vi "IMU AHRS Demo.vi"() -> ()   [LabVIEW 2014]
doc: "This example shows how to move a motor connected to an encoder and a wheel, and then read information about the system from an encoder.\n\nThis is an example of how to use feedback (from the encoder) to create an open loop system. If some control method was used, for example using PID, a closed loop system could be created."
uses:
  <vilib>/Rock Robotics/SystemInterfaces/i2clib/i2c_bus.ctl
  <vilib>/Platform/TimedLoop/XDataNode/timing_clust.ctl
  <vilib>/Platform/TimedLoop/XDataNode/nitl_modes.ctl
  <vilib>/Platform/TimedLoop/XDataNode/wakeup.ctl
  <vilib>/platform/TimedLoop/XDataNode/XDataNode.xnode
  <vilib>/Platform/TimedLoop/XDataNode/XDNodeRunTimeDep.lvlib
panel:
  out "R/P Alpha":dbl
  out "Yaw Alpha":dbl
  out "BadCal Mag":bool
  in  "I2C Bus":T1
  out "Anomaly":bool
  in  "Mag Set":T2={"Data Rate"=enum."220 Hz", "Range"=1, "Sense Enable"=TRUE, "Mag Scale"={"Xscale"=1.0, "Yscale"=1.0, "Zscale"=1.0}, "Mag Offset"={"Xzero"=0.0, "Yzero"=0.0, "Zzero"=0.0}, "Anomaly Thresh"=2.4, "Local Mag"=48.0} {"Range" items=["+/- 130 uT"=1, "+/- 190 uT"=2, "+/- 250 uT"=3, "+/- 400 uT"=4, "+/- 470 uT"=5, "+/- 560 uT"=6, "+/- 810 uT"=7]}
  out "Roll":cluster{dbl, dbl}(knob)={0.0, 152.0639793131716} scale=-180.0..180.0
  out "Pitch":cluster{dbl, dbl}(knob)={0.0, 152.0639793131716} scale=-90.0..90.0
  out "Yaw":cluster{dbl, dbl}(knob)={0.0, 152.0639793131716} scale=-180.0..180.0
  out "BadCal Accel":bool
  out "BadCal Gyro":bool
  in  "MagCal":bool=TRUE
  in  "Tilt Comp (Yaw)":bool
  out "Z Ang":dbl(graph)
  out "Z Mag":dbl(graph)
  out "Y Mag":dbl(graph)
  out "X Mag":dbl(graph)
  out "Y Ang":dbl(graph)
  out "X Ang":dbl(graph)
  out "FreeFall":bool
  out "Motion":bool
  out "Z acc":dbl(graph)
  out "Y acc":dbl(graph)
  out "X acc":dbl(graph)
  in  "tau acc (s)":dbl=0.047 format="%#_13g"
  in  "tau mag (s)":dbl=0.03 format="%#_13g"
  in  "Reset":bool
  in  "Accel Set":T3={"Data Rate"=enum."1.344 kHz", "Range"=0, "HPF Enable"=FALSE, "HPCF"=enum."00", "Sense Enable"=TRUE, "Accel Scale"={"Xscale"=1.0, "Yscale"=1.0, "Zscale"=1.0}, "Motion Thresh"=0.04} {"Range" items=["+/- 2 G", "+/- 4 G", "+/- 8 G", "+/- 16 G"]}
  in  "Gyro Set":T4={"Data Rate"=enum."800 Hz", "Range"=0, "HPF Enable"=FALSE, "HPCF"=enum."0000", "Sense Enable"=TRUE} {"Range" items=["+/- 245 deg/sec", "+/- 500 deg/sec", "+/- 2000 deg/sec"]}
  in  "Period (dt in ms)":i64=20
  out "Late?":bool
  # "FRC Team 836, The RoboBees: Sensor Fusion Demonstration / Designed for roboRIO\nDescription:\nThis series of Inertial Measurement Unit (IMU) subVIs is patterened after the WPI series for reading sensors, and includes several\nadditional IMU Application subVIs.  These application subVIs do the math required for sensor fusion, forming a basic Attitude\nand Heading Reference System (AHRS), with drift-free Roll, Pitch and Yaw outputs.  An IMU typically consists of a 3-axis \nAccelerometer, Rate Gyroscope, and Magnetometer (sometimes the Mag is absent, resulting in reduced capability).  Although\ntechnically incorrect, these devices are often referred to as 9 Degrees-of-Freedom (DoF) sensors (3 sensors with each 3\naxes in XYZ = 9 DoF). \n\nCompatible IMUs:\nThese IMU subVIs are designed to be used with the Adafruit 9-DoF IMU Breakout - containing L3GD20 (Gyro) + LSM303 \n(Accelerometer and Magnetometer) chips (Product ID: 1714), or the Adafruit 10-DoF IMU Breakout - whichs adds the BMP180\nchip (Product ID: 1604).  The 10-DoF IMU adds a Barometer for air temperature and pressure measurements (for indicating\naltitude, not attitude), and is not currently implemented.  The two IMU Application subVIs, COMPLE FILTER and TILT, are\nagnostic of IMU model, and compatible with separate sensors, as long as all sensor axes are aligned properly."
  # "AdaFruit 1714"
  # "Sensor Orientation:\nWhen Sensor oriented with positive X-axis\npointing forward, and positive Y-axis\npointing left, and positive Z axis pointing up :\n\nRoll is rotation about X-axis, clockwise roll,\n(looking in + X direction), is positive.\n\nPitch is rotation about Y-axis, clockwise pitch\n(looking in + Y direction), is positive.\n\nYaw is rotation about Z-axis, clockwise yaw\n(looking in + Z direction), is positive."
  # "RoboBees IMU and AHRS Demo Instructions:\n(1) Connect IMU to I2C port (4 wires: 5v/Gnd/SDA/SCK) on roboRIO.\n      Secure the IMU on Robot, orient as described at right.\n(2) Change the IP address of the roboRIO in the RoboBees IMU Demo project.\nYou can do this by right-clicking on RT CompactRIO Target in the project, selecting\nProperties, and modifying the IP Address setting in the General Category to match\nthat of your roboRIO.\n(3) Open Front Panel of the IMU OPEN subVI, you'll need that for step 8.\n(4) Establish Comm and Run this program (use Run Button deploy, not Build and deploy).\n(5) Follow the dialog boxes to perform Magnetometer Calibration.\n(6) Upon cal completion, observe Roll, Pitch, Yaw gauges as you (re)orient your sensor/robot.\n(7) Observe the 9 DoF display graphs for Gyro, Accel, and Mag in each XYZ axes.  The graphs are\n       useful in understanding how the sensor repsonds, but it's best to disable them once you no\n       longer need them, as they slow the dynamic response of the code under a Run button\n       deploy.  A simple way to do this is to wrap a Diagram Disable Structure (Structures Menu)\n       around the chart indicators on the Block Diagram. \n(8) Observe result of Magnetometer cal graph on the IMU OPEN front panel.  Use adjacent\n      graph display for reference.\n(9) If you don't like Mag cal result, repeat Mag cal by rerunning program.  See comments\nin IMU OPEN code for guidance.  If cal ok, stop program and load the 4 Mag cal\nparameters displayed in IMU OPEN (two each for X and Y axes), into Mag Set Cluster just below.\n(10) Set MagCal switch to false, then rerun this program.  This config is for competition.\n(11) Adjust the Loop Period as desired.  See implementation notes in IMU READ VI for guidance.\n(12) Adjust the Accelerometer tau and Magnetometer tau values as desired.  See implementation\n       notes in COMPLE FILTER VI  for guidance.\n(13) The Gyro/Accel cal process w/in IMU OPEN will auto-recal if it detects excessive\n        variation in the sample dataset, which likely indicates robot was bumped during cal.\n        Gently shake robot during program startup and observe BadCal indicators.\n(14) The roboRIO has two seperate I2C buses, On-Board and MXP.  This code works with the\n        On-Board I2C bus, but currently throws an error on the MXP I2C bus, tested with a Rev\n        Robotics expansion board.  \n\nPls provide attribution to FRC Team 836, The RoboBees if you find this useful !!"
  # "Robot\nFront"
  # "Loop Timing can affect operation"
  # "roboRIO I2C    DIO-0  V     Gnd    SCL     SDA"
  # "Note that Period (dt) can probably be reduced to less than 20 ms before Timed Loop starts running late, in this demo, since it's the only code running.  Using these IMU VIs in your code, however, may require a longer loop period to allow the CPU time to execute your other robot code  - you can use the same technique of adjusting the period while monitoring the Late indicator for optimization when you integrate these VIs into your code.  You can disable the 9 DoF graphs to considerably improve speed of code (when deployed with the Run button), in which case Period can be much lower (~3 ms, again, provided this is the only code running).  Benchmark was against 2015 roboRIO."
  # "Sensor Fusion Design:"
  # "Sensor Fusion Settings"
  # "Adjust these tau settings to optimize the sensor fusion.  tau acc affects\nRoll and Pitch.  tau mag affects Yaw.   Consider that alpha = tau / (tau + dt),\nand that alpha is what affects the fusion performance.  An alpha of about 0.7 for\nRoll and Pitch, and an alpha of about 0.6 for Yaw appear to be good starting points."
  # "Red needles are filtered AHRS readings.  Grey needles are raw Gyro readings.\nGrey needles will drift.  With proper tau settings, red needles will not drift.\nThat's the power of sensor fusion ..."
  # "Enabling this corrects Yaw error when Pitch and Roll are\nnon-zero, however, Yaw will be affected by Accelerometer\nmovement and noise.  Reference IMU Comple Filter subVI\nnotes for more insight on this tradeoff."
  # "Gyro"
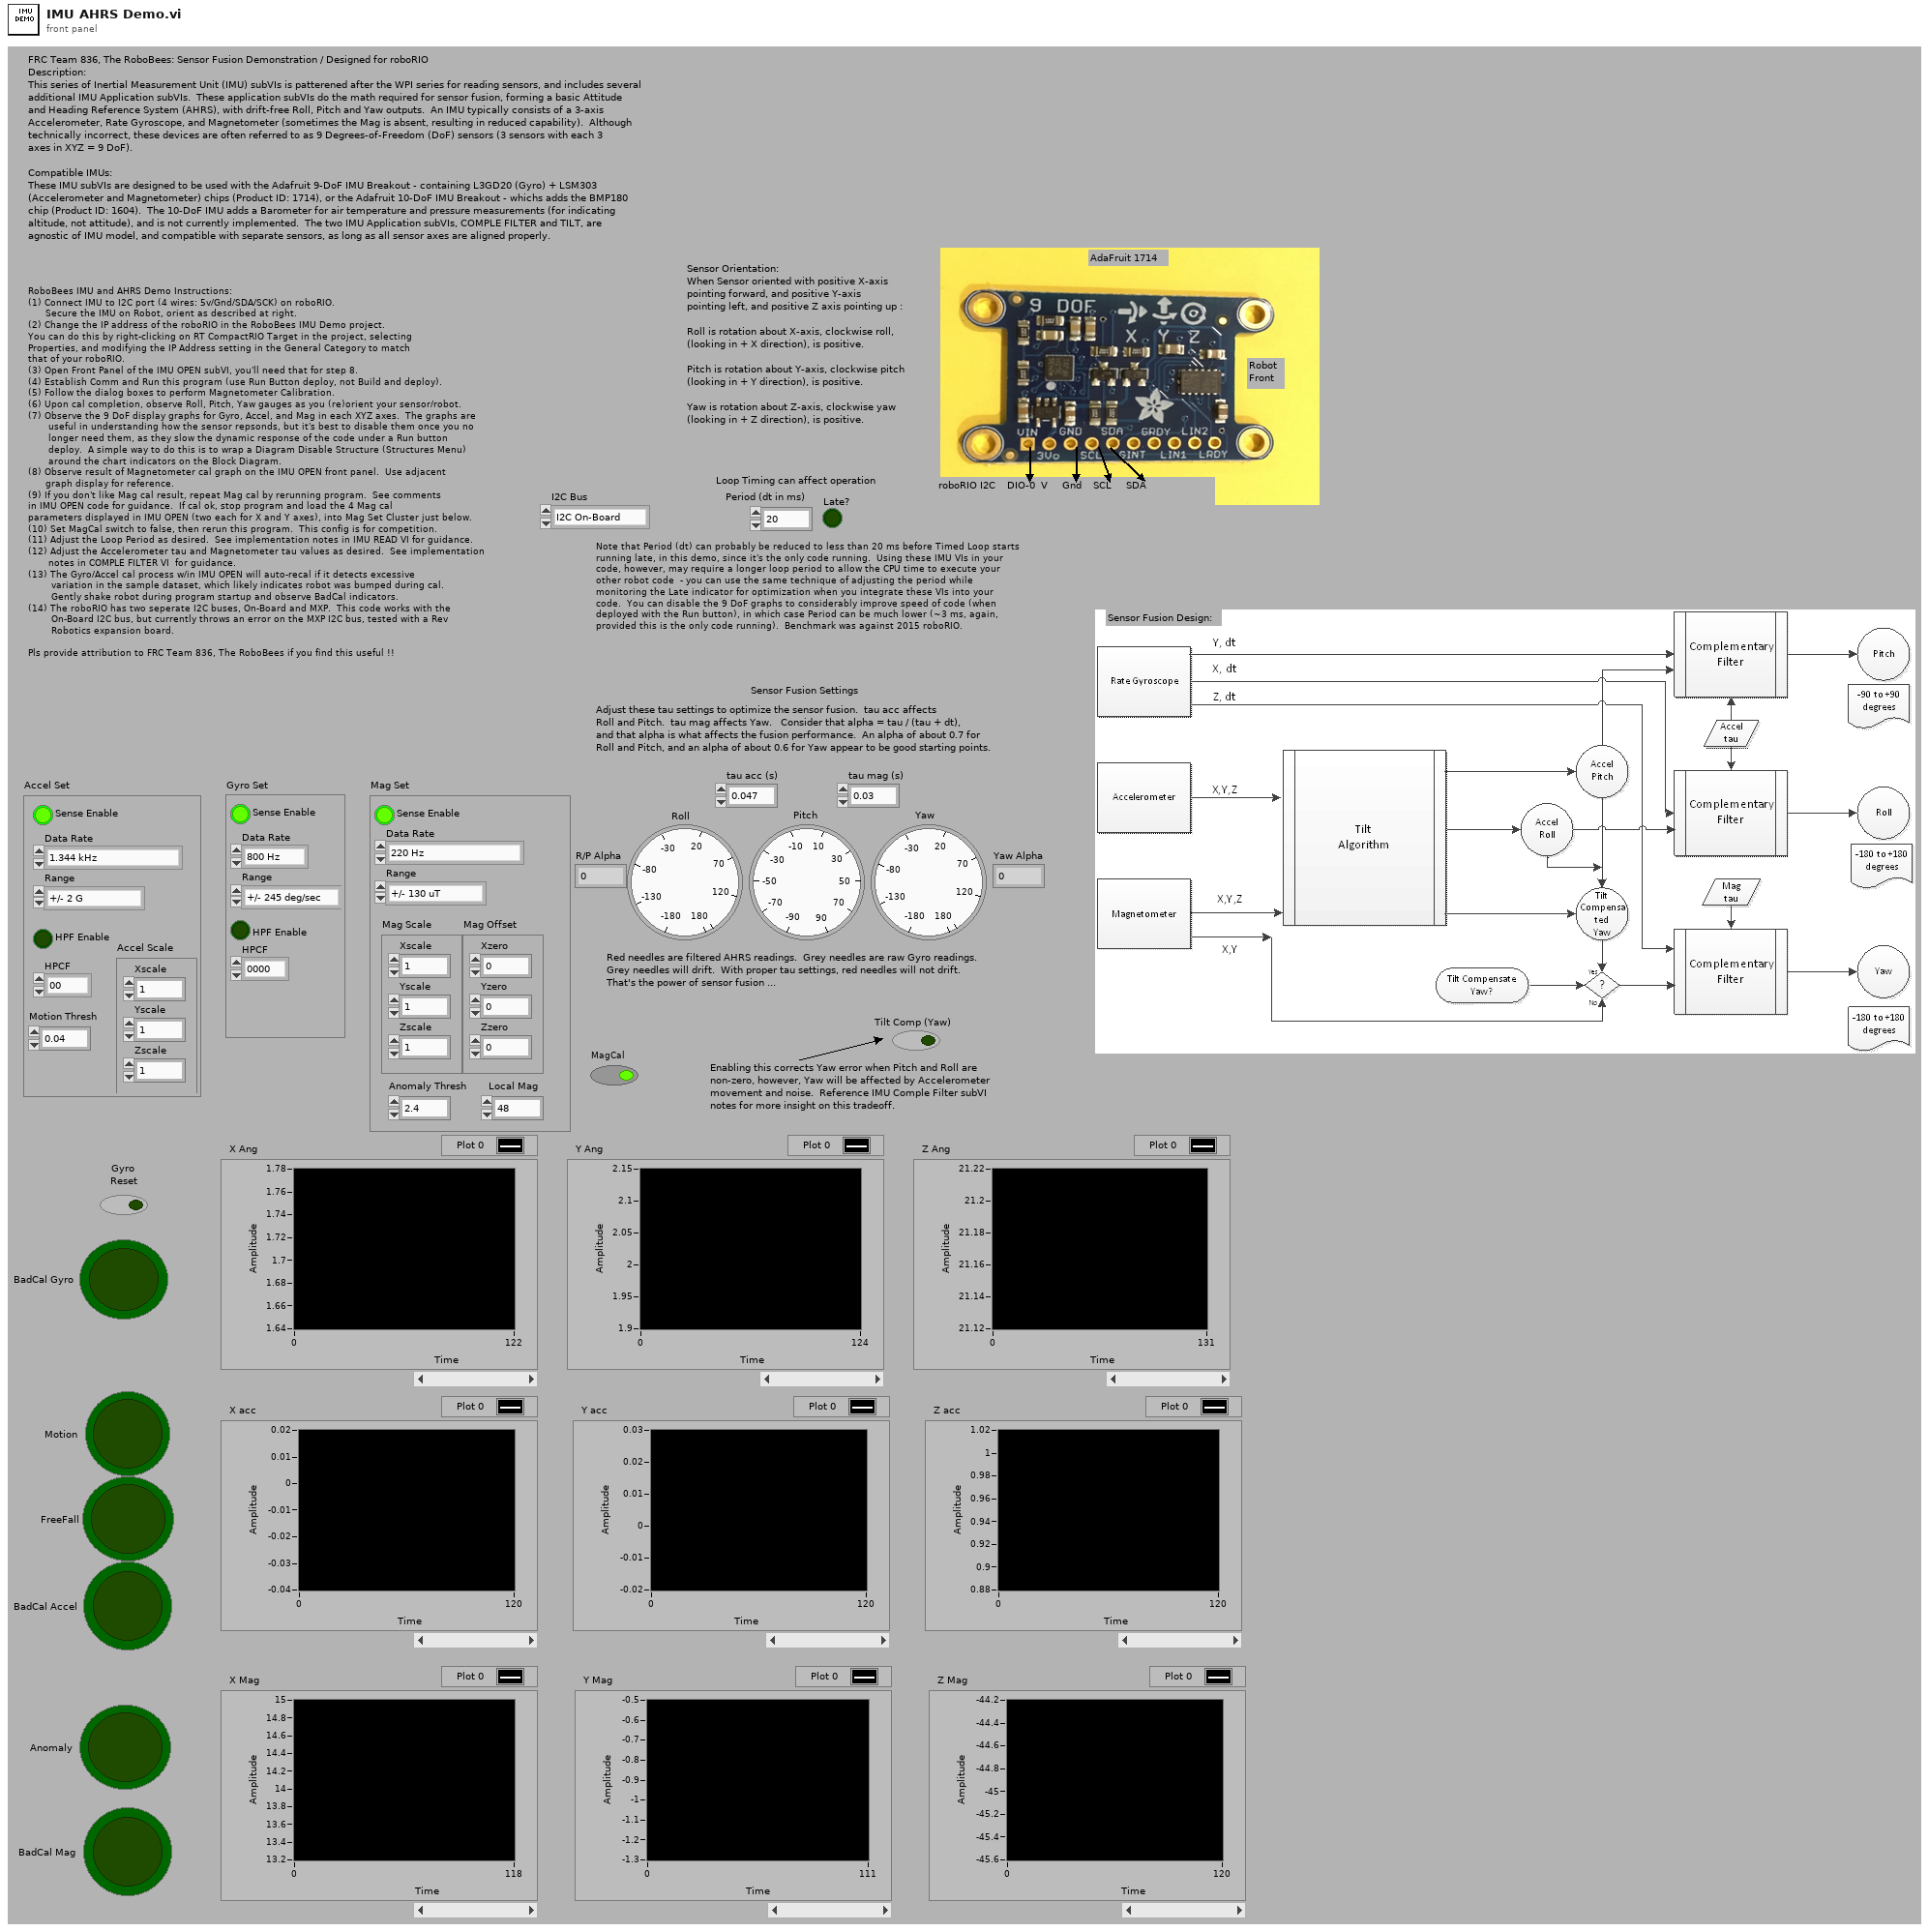
[diagram p1: front panel]
types:
  T1 = typedef "i2c_bus.ctl" = enum16{"I2C On-Board", "I2C MXP", "Invalid"}
  T2 = cluster{"Data Rate":enum8{"0.75 Hz", "1.5 Hz", "3.0 Hz", "7.5 Hz", "15 Hz", "30 Hz", "75 Hz", "220 Hz"}, "Range":u8, "Sense Enable":bool, "Mag Scale":cluster{"Xscale":dbl, "Yscale":dbl, "Zscale":dbl}, "Mag Offset":cluster{"Xzero":dbl, "Yzero":dbl, "Zzero":dbl}, "Anomaly Thresh":dbl, "Local Mag":dbl}
  T3 = cluster{"Data Rate":enum8{"Power-down mode", "1 Hz", "10 Hz", "25 Hz", "50 Hz", "100 Hz", "200 Hz", "400 Hz", "Low-power mode only", "1.344 kHz"}, "Range":u8, "HPF Enable":bool, "HPCF":enum8{"00", "01", "10", "11"}, "Sense Enable":bool, "Accel Scale":cluster{"Xscale":dbl, "Yscale":dbl, "Zscale":dbl}, "Motion Thresh":dbl}
  T4 = cluster{"Data Rate":enum8{"100 Hz", "200 Hz", "400 Hz", "800 Hz"}, "Range":u8, "HPF Enable":bool, "HPCF":enum8{"0000", "0001", "0010", "0011", "0100", "0101", "0110", "0111", "1000", "1001"}, "Sense Enable":bool}
  T5 = cluster{"BadCal Gyro":bool, "BadCal Accel":bool, "BadCal Mag":bool}
  T6 = typedef "IMUDevRef.ctl" = cluster{"DevStatus":errorcluster, "Gyro Address":u8, "Gyro Range":u8, "Mean Rates":cluster{"Xmo":dbl, "Ymo":dbl, "Zmo":dbl}, "StdDev Rates":cluster{"Xsdo":dbl, "Ysdo":dbl, "Zsdo":dbl}, "Fast":bool, "Reset":bool, "Accel Address":u8, "Accel Range":u8, "Accel Scale":cluster{"Xscale":dbl, "Yscale":dbl, "Zscale":dbl}, "Mag Address":u8, "Mag Range":u8, "G Sense":bool, "A Sense":bool, "M Sense":bool, "Accel Offset":cluster{"Xzero":dbl, "Yzero":dbl, "Zzero":dbl}, "Motion Thresh":dbl, "Mag Scale":cluster{"Xscale":dbl, "Yscale":dbl, "Zscale":dbl}, "Mag Offset":cluster{"Xzero":dbl, "Yzero":dbl, "Zzero":dbl}, "I2C Bus":T1, "Handle":i32, "Controller":T7, "Anomaly Thresh":dbl, "Local Mag":dbl}
  T7 = typedef "FPGA_TypedefDigitalModule.ctl" = enum16{"Digital Module 1", "Digital Module 2"}
  T8 = typedef "XDNodeRunTimeDep.lvlib/timing_clust.ctl" = cluster{"Expected End [f-1]":u64, "Actual End [f-1]":u64, "Finished Late? [f-1]":bool, "Expected End [i-1]":u64, "Actual End [i-1]":u64, "Finished Late? [i-1]":bool, "Expected Start [i]":u64, "Actual Start [i]":u64, "Expected Start [f]":u64, "Actual Start [f]":u64, "Source Name":string, "Structure Name":string, "Period":i64, "Deadline":i64, "Offset":i64, "Start":i64, "Priority":i32, "Timeout":i32, "Mode":T9, "Wakeup Reason":T10, "Error":errorcluster, "Source Type":string, "Secondary Source Type":string, "Global End Time":u64, "Global Start Time":u64, "Frame Duration":u64, "Iteration Duration":u64, "Assigned CPU":i32, "I/O Scan Engine Mode":u32}
  T9 = typedef "XDNodeRunTimeDep.lvlib/nitl_modes.ctl" = enum32{"No Change", "Process missed periods, maintain original phase", "Discard missed periods, maintain original phase", "Process missed periods, ignore original phase", "Discard missed periods, ignore original phase"}
  T10 = typedef "XDNodeRunTimeDep.lvlib/wakeup.ctl" = enum32{"Normal", "Aborted", "Asynchronous wakeup", "Timing source error", "Timed loop error", "Timeout"}
  T11 = typedef "Gyro.ctl" = cluster{"Xrate":dbl, "Yrate":dbl, "Zrate":dbl, "Xdeg":dbl, "Ydeg":dbl, "Zdeg":dbl, "dt":dbl}
  T12 = typedef "Accel.ctl" = cluster{"Xaccel":dbl, "Yaccel":dbl, "Zaccel":dbl, "Motion":bool, "Threshold":dbl, "FreeFall":bool}
  T13 = typedef "Mag.ctl" = cluster{"Xmag":dbl, "Ymag":dbl, "Zmag":dbl, "Anomaly":bool}
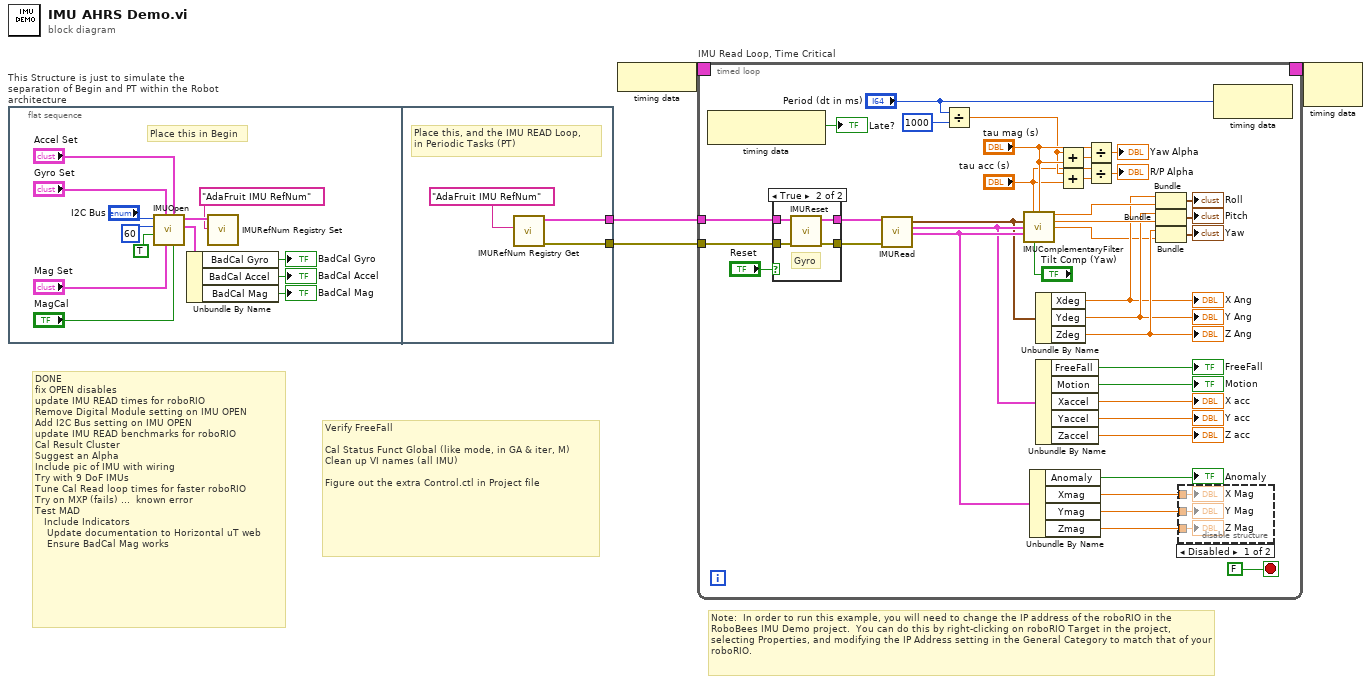
[diagram p0: block diagram]
diagram:
  # "DONE\nfix OPEN disables\nupdate IMU READ times for roboRIO\nRemove Digital Module setting on IMU OPEN\nAdd I2C Bus setting on IMU OPEN\nupdate IMU READ benchmarks for roboRIO\nCal Result Cluster\nSuggest an Alpha\nInclude pic of IMU with wiring\nTry with 9 DoF IMUs\nTune Cal Read loop times for faster roboRIO\nTry on MXP (fails) ...  known error\nTest MAD\n   Include Indicators\n    Update documentation to Horizontal uT web\n    Ensure BadCal Mag works"
  # "Verify FreeFall\n\nCal Status Funct Global (like mode, in GA & iter, M) \nClean up VI names (all IMU)\n\nFigure out the extra Control.ctl in Project file"
  # "Note:  In order to run this example, you will need to change the IP address of the roboRIO in the RoboBees IMU Demo project.  You can do this by right-clicking on roboRIO Target in the project, selecting Properties, and modifying the IP Address setting in the General Category to match that of your roboRIO."
  n1 = flat-sequence "This Structure is just to simulate the separation of Begin and PT within the Robot architecture" {
    tunnel: [w19] -> w2
    tunnel: [w18] -> w1
    frame #0 {
      # "Place this in Begin"
      n2 = call "IMUOpen.vi"("MagCal"="MagCal", "Accel Set"="Accel Set", "Mag Set"="Mag Set", "Gyro Set"="Gyro Set", "Fast"=TRUE, "CalSamples"=60 ("CalAvg"), "I2C Bus"="I2C Bus") -> ("Cal Result"=w8:T5, "AdaIMUDevRef Out"=w15:T6)  [unwired: 2 in, 1 out]
      n3 = Unbundle By Name(w8) -> ("BadCal Gyro"=→"BadCal Gyro":bool, "BadCal Accel"=→"BadCal Accel":bool, "BadCal Mag"=→"BadCal Mag":bool)
      n4 = call "IMURefNum Registry Set.vi"("refnum name"="AdaFruit IMU RefNum", "AdaIMUDevRef"=w15) -> ()  [unwired: 8 in, 2 out]
    }
    frame #1 {
      # "Place this, and the IMU READ Loop,\nin Periodic Tasks (PT)"
      n5 = call "IMURefNum Registry Get.vi"("refnum name"="AdaFruit IMU RefNum") -> ("error out"=w18:errorcluster, "AdaIMUDevRef Out"=w19:T6)  [unwired: 9 in]
    }
  }
  n6 = node-c288() -> (w4:T8)
  n7 = timed-loop "IMU Read Loop, Time Critical" {
    timing: w4 -> [_]
    timing-out: [_] -> w3
    tunnel: w2 -> [w52]
    tunnel: w1 -> [w51]
    stop <- FALSE stop-if-true
    n8 = node-c288() -> (→"Late?":bool)  [unwired: 1 in]
    n9 = case shown="True" "Reset" {
      tunnel: w52 -> [w63 w67]
      tunnel: [w63 w66] -> w56
      tunnel: [w62 w65] -> w55
      tunnel: w51 -> [w62 w64]
      frame False {
      }
      frame True {
        # "Gyro"
        n10 = call "IMUReset.vi"("error in (no error)"=w64, "AdaIMUDevRef"=w67) -> ("error out"=w65:errorcluster, "AdaIMUDevRef Out"=w66:T6)  [unwired: 8 in]
      }
    }
    n11 = call "IMURead.vi"("AdaIMUDevRef"=w56, "error in"=w55) -> ("Gyro"=w32:T11, "Accel"=w33:T12, "Mag"=w45:T13)  [unwired: 9 in, 2 out]
    n12 = Divide(x="Period (dt in ms)", y=i64 1000) -> (x/y=w23:dbl)
    n13 = call "IMUComplementaryFilter.vi"("tau acc"="tau acc (s)", "tau mag"="tau mag (s)", "Gyro"=w32, "Accel"=w33, "Mag"=w45, "Tilt Comp (Yaw)"="Tilt Comp (Yaw)") -> ("Roll"=w39:dbl, "Pitch"=w40:dbl, "Yaw"=w30:dbl)  [unwired: 7 in]
    n14 = Unbundle By Name(w45) -> ("Anomaly"=→"Anomaly":bool, "Xmag"=w44:dbl, "Ymag"=w43:dbl, "Zmag"=w42:dbl)
    n15 = Unbundle By Name(w32) -> ("Xdeg"=w36:dbl, "Ydeg"=w37:dbl, "Zdeg"=w38:dbl)
    "X Ang" <- w36
    "Y Ang" <- w37
    "Z Ang" <- w38
    n16 = Unbundle By Name(w33) -> ("FreeFall"=→"FreeFall":bool, "Motion"=→"Motion":bool, "Xaccel"=→"X acc":dbl, "Yaccel"=→"Y acc":dbl, "Zaccel"=→"Z acc":dbl)
    n17 = Add(x=w23, y="tau mag (s)") -> (x+y=w29:dbl)
    n18 = Add(x=w23, y="tau acc (s)") -> (x+y=w27:dbl)
    n19 = Divide(x="tau mag (s)", y=w29) -> (x/y=→"Yaw Alpha":dbl)
    n20 = Divide(x="tau acc (s)", y=w27) -> (x/y=→"R/P Alpha":dbl)
    n21 = Bundle("Xdeg"=w36, "Roll"=w39) -> (→"Roll":cluster{"Xdeg":dbl, "Roll":dbl})  [unwired: 1 in]
    n22 = Bundle("Ydeg"=w37, "Pitch"=w40) -> (→"Pitch":cluster{"Ydeg":dbl, "Pitch":dbl})  [unwired: 1 in]
    n23 = Bundle("Zdeg"=w38, "Yaw"=w30) -> (→"Yaw":cluster{"Zdeg":dbl, "Yaw":dbl})  [unwired: 1 in]
    n24 = disable-structure shown="Disabled" {
      disable-tunnel: w44 -> [w61 _]
      disable-tunnel: w43 -> [w60 _]
      disable-tunnel: w42 -> [w59 _]
      frame Disabled {
        "Z Mag" <- w59
        "X Mag" <- w61
        "Y Mag" <- w60
      }
      frame Enabled {
      }
    }
    n25 = node-c288("Period (dt in ms)") -> ()  [unwired: 1 out]
  }
  n26 = node-c288(w3) -> ()  [unwired: 1 out]
